vi "NISE.local.Unreserve.vi"(0 "SLSC Local in":refnum<class "SLSC Interface.lvclass">, 5 "devices":refnum<k21>="$DefaultDevices", 11 "error in (no error)":errorcluster) -> (4 "SLSC Local out":refnum<class "SLSC Interface.lvclass">, 15 "error out":errorcluster)   [LabVIEW 2016, in "SLSC Interface.lvclass"]
uses:
  SLSC Interface Class/SLSC Interface.lvclass
  SLSC Interface Class/NISE.Read session.vi
  SLSC Interface Class/NISE.Write session.vi
  <vilib>/SLSC/SLSC.lvlib
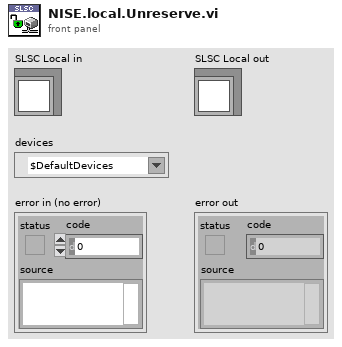
[diagram p1: front panel]
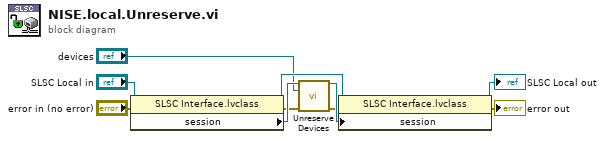
[diagram p0: block diagram]
diagram:
  n1 = property class="SLSC Interface.lvclass"(reference="SLSC Local in", error in="error in (no error)") -> (reference out=w9:refnum<class "SLSC Interface.lvclass">, error out=w6:errorcluster, "session"=w7:refnum<k21>)
  n2 = call <vilib>:"Unreserve Devices.vi"("session in"=w7, "devices"="devices", "error in (no error)"=w6) -> ("session out"=w5:refnum<k21>, "error out"=w4:errorcluster)  [unwired: 11 in]
  n3 = property class="SLSC Interface.lvclass"(reference=w9, error in=w4, "session"=w5) -> (reference out=→"SLSC Local out":refnum<class "SLSC Interface.lvclass">, error out=→"error out":errorcluster)
